vi "thinned_image_to_centerline.vi"(3 "error in":errorcluster, 4 "Temp Image":T1, 5 "Skeleton Image":T1) -> (0 "error out":errorcluster, 1 "Algorithm timed out":bool, 2 "Centline Pixels":i32[][](array[numeric]))   [LabVIEW 2019]
uses:
  <vilib>/vision/Image Controls.llb/IMAQ Image.ctl
  a49f2ef7-d53c-4424-bee3-5857753b5dab.vi
  iterative_segments_to_centerline_oneiteration.vi
  <vilib>/vision/NI_Vision_Development_Module.lvlib
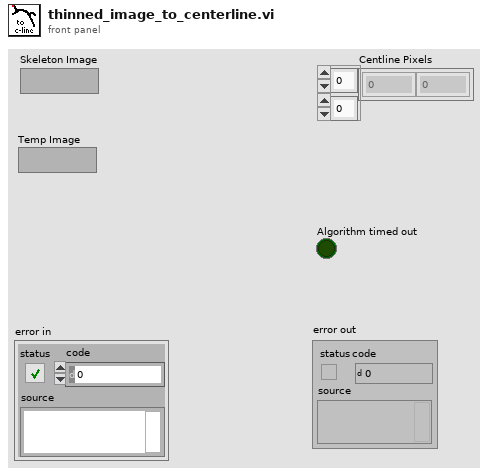
[diagram p1: front panel]
types:
  T1 = typedef "IMAQ Image.ctl" = refnum<image>
  T2 = enum32{"AutoM", "Close", "Dilate", "Erode", "Gradient", "Gradient out", "Gradient in", "Hit miss", "Open", "PClose", "POpen", "Thick", "Thin"}
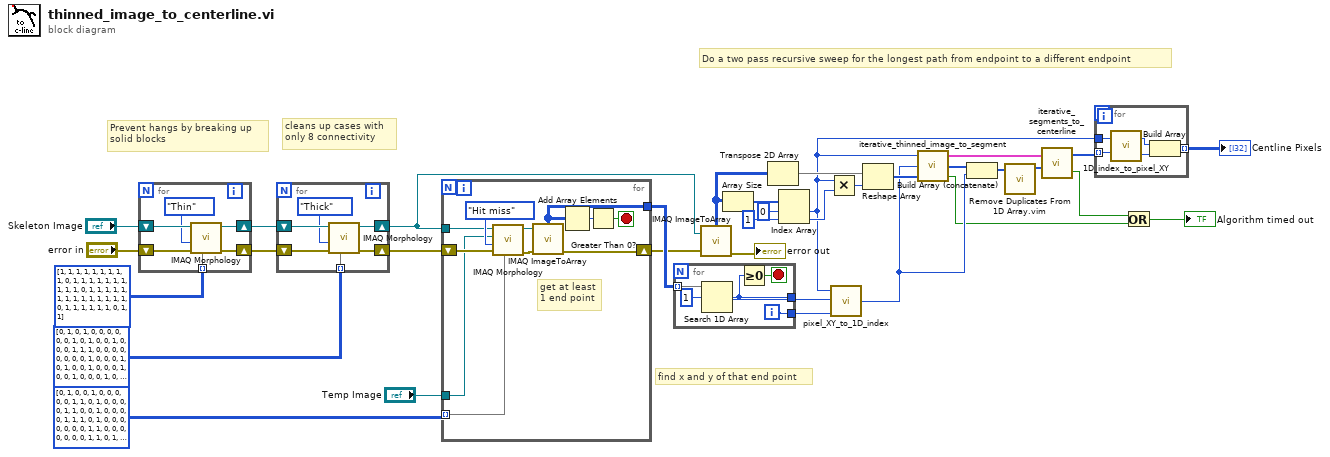
[diagram p0: block diagram]
diagram:
  # "cleans up cases with \nonly 8 connectivity"
  # "Prevent hangs by breaking up\nsolid blocks"
  # "find x and y of that end point"
  # "Do a two pass recursive sweep for the longest path from endpoint to a different endpoint"
  n1 = for {
    shift-right: [w39] -> w5
    shift-left: "error in" -> [w40]
    shift-right: [w37] -> w3
    shift-left: "Skeleton Image" -> [w38]
    tunnel: i32[][][] [[[1, 1, 1], [1, 1, 1], [1, 1, 1]], [[0, 1, 1], [1, 1, 1], [1, 1, 1]], [[1, 1, 0], [1, 1, 1], [1, 1, 1]], [[1, 1, 1], [1, 1, 1], [1, 1, 0]], [[1, 1, 1], [1, 1, 1], [0, 1, 1]]] ("End Point Structural Element") -> [w35] mode=indexing
    n2 = call "IMAQ Morphology"("Structuring Element"=w35, "error in (no error)"=w40, "Operation"=T2."Thin", "Image Src"=w38) -> ("error out"=w39:errorcluster, "Image Dst Out"=w37:T1)  [unwired: 6 in]
  }
  n3 = for {
    shift-right: [w45] -> w4
    shift-left: w5 -> [w46]
    shift-right: [w43] -> w2
    shift-left: w3 -> [w44]
    tunnel: i32[][][] [[[0, 1, 0], [1, 0, 0], [0, 0, 0]], [[0, 1, 0], [1, 0, 0], [1, 0, 0]], [[0, 1, 1], [1, 0, 0], [0, 0, 0]], [[0, 0, 0], [1, 0, 0], [0, 1, 0]], [[1, 0, 0], [1, 0, 0], [0, 1, 0]], [[0, 1, 0], [0, 0, 1], [0, 0, 0]], [[0, 1, 0], [0, 0, 1], [0, 0, 1]], [[1, 1, 0], [0, 0, 1], [0, 0, 0]], [[0, 0, 0], [1, 0, 0], [0, 1, 1]], [[0, 0, 0], [0, 0, 1], [0, 1, 0]], [[0, 0, 1], [0, 0, 1], [0, 1, 0]]] ("Enumerated Structuring Elements") -> [w41] mode=indexing
    n4 = call "IMAQ Morphology"("Structuring Element"=w41, "error in (no error)"=w46, "Operation"=T2."Thick", "Image Src"=w44) -> ("error out"=w45:errorcluster, "Image Dst Out"=w43:T1)  [unwired: 6 in]
  }
  n5 = for {
    shift-right: [w52] -> w18
    shift-left: w4 -> [w56]
    tunnel: i32[][][] [[[0, 1, 0], [0, 1, 0], [0, 0, 0]], [[0, 1, 1], [0, 1, 0], [0, 0, 0]], [[1, 1, 0], [0, 1, 0], [0, 0, 0]], [[1, 1, 1], [0, 1, 0], [0, 0, 0]], [[0, 0, 0], [1, 1, 0], [0, 0, 0]], [[0, 0, 0], [1, 1, 0], [1, 0, 0]], [[1, 0, 0], [1, 1, 0], [0, 0, 0]], [[1, 0, 0], [1, 1, 0], [1, 0, 0]], [[0, 0, 0], [0, 1, 0], [0, 1, 0]], [[0, 0, 0], [0, 1, 0], [0, 1, 1]], [[0, 0, 0], [0, 1, 0], [1, 1, 0]], [[0, 0, 0], [0, 1, 0], [1, 1, 1]], [[0, 0, 0], [0, 1, 1], [0, 0, 0]], [[0, 0, 0], [0, 1, 1], [0, 0, 1]], [[0, 0, 1], [0, 1, 1], [0, 0, 0]], [[0, 0, 1], [0, 1, 1], [0, 0, 1]]] ("End Point Structural Element") -> [w55] mode=indexing
    tunnel: "Temp Image" -> [w48]
    tunnel: [w49] -> w20
    tunnel: w2 -> [w47]
    stop <- w50 stop-if-true
    # "get at least\n1 end point"
    n6 = call "IMAQ Morphology"("Structuring Element"=w55, "error in (no error)"=w56, "Operation"=T2."Hit miss", "Image Dst"=w48, "Image Src"=w47) -> ("error out"=w54:errorcluster, "Image Dst Out"=w53:T1)  [unwired: 5 in]
    n7 = call "IMAQ ImageToArray"("error in (no error)"=w54, "Image"=w53) -> ("error out"=w52:errorcluster, "Image Pixels (U8)"=w49:u8[][])  [unwired: 2 in, 3 out]
    n8 = Add Array Elements(numeric array=w49) -> (sum=w51:u8)
    n9 = Greater Than 0?(x=w51) -> (x > 0?=w50:bool)
  }
  n10 = for {
    tunnel: w20 -> [w62] mode=indexing
    tunnel: [w59] -> w16
    tunnel: [w58] -> w15
    i -> [w58]
    stop <- w60 stop-if-true
    n11 = Search 1D Array(1D array=w62, element=u8 1) -> (index of element=w59:i32)  [unwired: 1 in]
    n12 = Greater Or Equal To 0?(x=w59) -> (x >= 0?=w60:bool)
  }
  n13 = call "IMAQ ImageToArray"("error in (no error)"=w18, "Image"=w2) -> ("error out"=→"error out":errorcluster, "Image Pixels (U8)"=w17:u8[][])  [unwired: 2 in, 3 out]
  n14 = Array Size(array=w17) -> (size(s)=w34:i32[])
  n15 = Transpose 2D Array(2D array=w17) -> (transposed array=w29:u8[][])
  n16 = Index Array(array=w34, index #1=0 ("index"), index #2=1 ("index")) -> (element #1=w22:i32, element #2=w30:i32)
  n17 = Multiply(x=w22, y=w30) -> (x*y=w31:i32)
  n18 = call "pixel_XY_to_1D_index.vi"("Y"=w15, "X"=w16, "Image Height"=w22) -> ("ID Index"=w26:i32)
  n19 = Reshape Array(w29, w31) -> (w28:u8[])
  n20 = call "iterative_thinned_image_to_segment.vi"("1D image array"=w28, "Segment Start Idx"=w26, "Image Height"=w22) -> ("Algorithm timed out"=w11:bool, "Endpoints"=w27:i32[], "Segment Sequence Cluster Arrays"=w21:cluster{i32[]}[])
  n21 = Build Array (concatenate)(w27, w26) -> (w25:i32[])
  n22 = call "Remove Duplicates From 1D Array.vim"("array"=w25) -> ("array with duplicates removed"=w24:i32[])  [unwired: 10 in]
  n23 = call "iterative_segments_to_centerline.vi"("Endpoints"=w24, "Segment Sequence Cluster Arrays"=w21) -> ("Timed Out"=w12:bool, "Best Centerline 1D"=w23:i32[])
  n24 = for {
    tunnel: w23 -> [w67] mode=indexing
    tunnel: w22 -> [w66]
    tunnel: [w63] -> w13 mode=indexing
    n25 = call "1D_index_to_pixel_XY.vi"("ID Index"=w67, "Image Height"=w66) -> ("Y"=w64:i32, "X"=w65:i32)
    n26 = Build Array(w65, w64) -> (w63:i32[])
  }
  "Centline Pixels" <- w13
  n27 = Or(x=w12, y=w11) -> (x .or. y?=→"Algorithm timed out":bool)
